vi "calculate edge fit.vi"(8 "error in (no error)":errorcluster, 11 "LineCCD in":refnum<class "LineCCD.lvclass">) -> (0 "error out":errorcluster, 3 "LineCCD out":refnum<class "LineCCD.lvclass">)   [LabVIEW 2012, in "LineCCD.lvclass"]
uses:
  LineCCD.lvclass
  LineCCD.lvclass/LineCCD.ctl
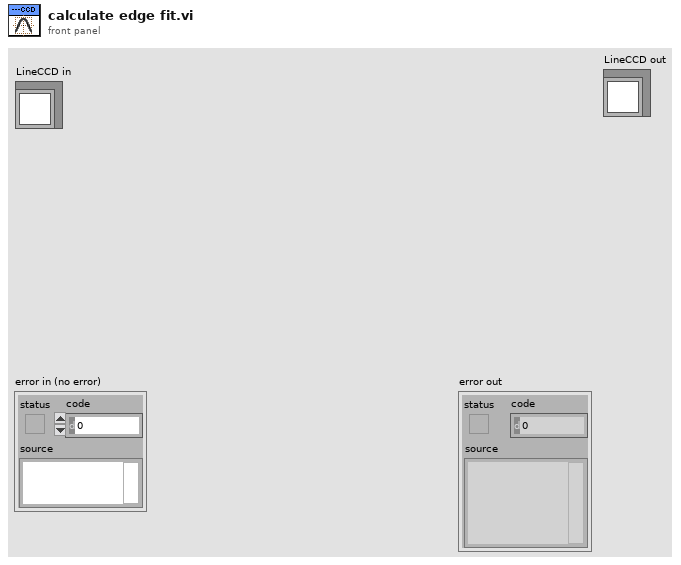
[diagram p1: front panel]
types:
  T1 = typedef "LineCCD.lvclass/fitting parameters.ctl" = cluster{"y_min":dbl, "y_mean":dbl, "A_g":dbl, "STD":dbl, "x_0":dbl}
  T2 = cluster{"best fit parameters[0]":dbl, "best fit parameters[1]":dbl, "best fit parameters[2]":dbl, "best fit parameters[3]":dbl, "best fit parameters[4]":dbl}
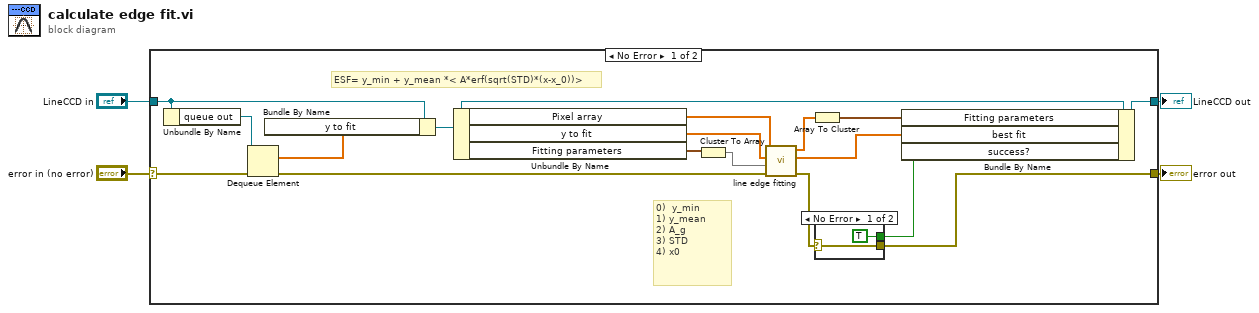
[diagram p0: block diagram]
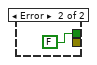
[diagram p2: hidden frame]
diagram:
  n1 = case shown="No Error" "error in (no error)" {
    selector: "error in (no error)" -> [w19 w26]
    tunnel: [w6 w26] -> w3
    tunnel: [w21 w25] -> w1
    tunnel: "LineCCD in" -> [w17 w25]
    frame No Error {
      # "ESF= y_min + y_mean *< A*erf(sqrt(STD)*(x-x_0))>"
      # "0)  y_min\n1) y_mean\n2) A_g\n3) STD\n4) x0"
      n2 = Unbundle By Name(w17) -> ("queue out"=w20:refnum<queue>)
      n3 = Dequeue Element(queue=w20, error in (no error)=w19) -> (element=w12:dbl[], error out=w18:errorcluster)  [unwired: 1 in, 2 out]
      n4 = Bundle By Name(cluster=w17, "y to fit"=w12) -> (w16:refnum<class "LineCCD.lvclass">)
      n5 = Unbundle By Name(w16) -> ("Pixel array"=w14:dbl[], "y to fit"=w13:dbl[], "Fitting parameters"=w11:T1)
      n6 = Cluster To Array(cluster=w11) -> (array=w10:dbl[])
      n7 = call "line edge fitting.vi"("error in (no error)"=w18, "Paramter guess"=w10, "y"=w13, "x"=w14) -> ("error out"=w7:errorcluster, "best nonlinear fit"=w15:dbl[], "best fit parameters"=w9:dbl[])  [unwired: 4 in, 1 out]
      n8 = Array To Cluster(array=w9) -> (cluster=w8:T2)
      n9 = case shown="No Error" w7 {
        selector: w7 -> [w23 _]
        tunnel: [w23 _] -> w6
        tunnel: [TRUE FALSE] -> w5
        frame No Error {
        }
        frame Error {
        }
      }
      n10 = Bundle By Name(cluster=w16, "Fitting parameters"=w8, "best fit"=w15, "success?"=w5) -> (w21:refnum<class "LineCCD.lvclass">)
    }
    frame Error {
    }
  }
  "error out" <- w3
  "LineCCD out" <- w1
